vi "Test AF Stratification.vi"() -> ()   [LabVIEW 2020]
uses:
  CoolApp/CoolApp.lvclass
  C:/Program Files (x86)/National Instruments/LabVIEW 2020/vi.lib/ActorFramework/Actor/Actor.lvclass
  <vilib>/ActorFramework/Actor/Actor.lvclass
panel:
  out "error out":errorcluster
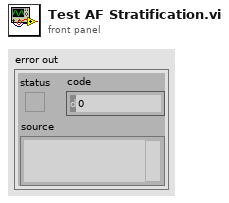
[diagram p1: front panel]
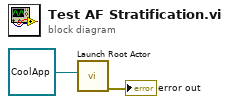
[diagram p0: block diagram]
diagram:
  n1 = call <vilib>:"Launch Root Actor.vi"("Actor"=refnum<class "CoolApp.lvclass"> refnum ("LAF2024Q2.lvlib:CoolApp.lvclass")) -> ("error out"=→"error out":errorcluster)  [unwired: 9 in, 1 out]
